vi "FRIC_navX_Get_RawValues_GyroAccelMag.vi"(5 "Device Number":T1, 7 "Update":bool) -> (2 "Raw Values (out)":T2)   [LabVIEW 2016, in "navX Library.lvlib"]
doc: "This navX VI returns the raw values from the Gyro, Accel, and Mag sensors."
uses:
  navX Library.lvlib
  _TypeDefs/FRIC_navX_DeviceNumbersTypeDef.ctl
  _TypeDefs/Z900_navX_DeviceRegisters.ctl
  _Util/Z900_navX_Util_LittleEndian_to_BigEndian.vi
  _Internal/FRIC_navX_Get_Registry.vi
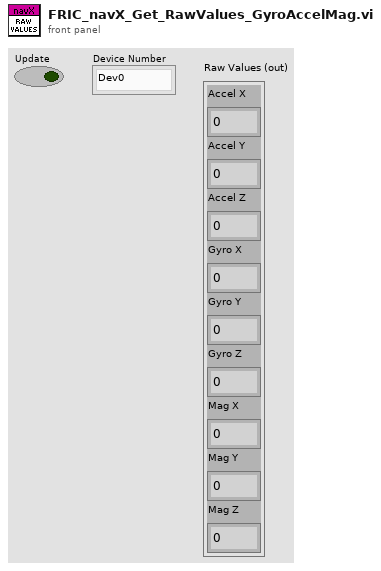
[diagram p1: front panel]
types:
  T1 = typedef "navX Library.lvlib/FRIC_navX_DeviceNumbersTypeDef.ctl" = enum16{"Dev0", "Dev1", "Dev2", "Dev3"}
  T2 = cluster{"Accel X":dbl, "Accel Y":dbl, "Accel Z":dbl, "Gyro X":dbl, "Gyro Y":dbl, "Gyro Z":dbl, "Mag X":dbl, "Mag Y":dbl, "Mag Z":dbl}
  T3 = typedef "navX Library.lvlib/Z900_navX_DeviceRegisters.ctl" = u8
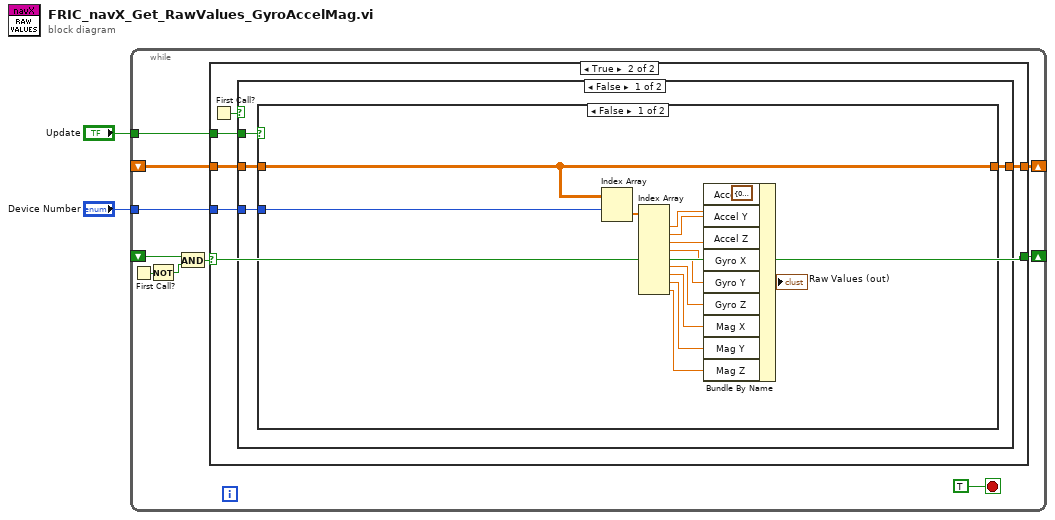
[diagram p0: block diagram]
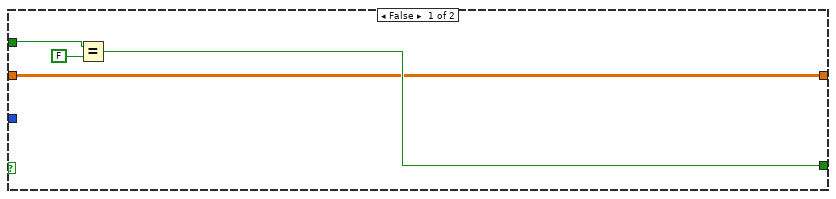
[diagram p2: hidden frame]
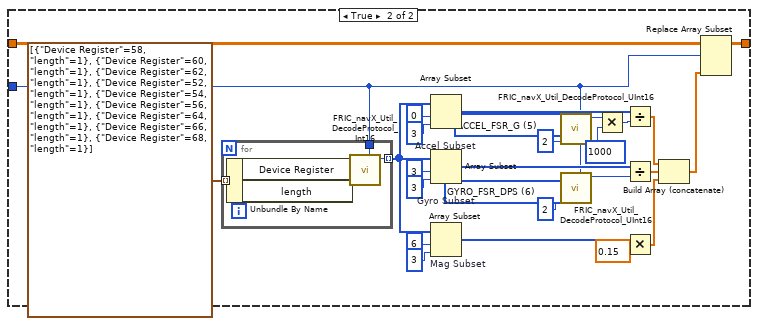
[diagram p3: hidden frame]
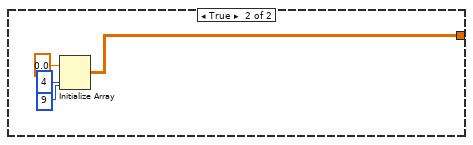
[diagram p4: hidden frame]
diagram:
  n1 = while {
    shift-right: [w12] -> _
    shift-left: _ -> [w9]
    tunnel: "Update" -> [w10]
    tunnel: "Device Number" -> [w8]
    shift-right: [w3] -> _
    shift-left: _ -> [w4]
    stop <- TRUE stop-if-true
    n2 = First Call?() -> (First Call?: T/F=w6:bool)
    n3 = Not(x=w6) -> (.not. x?=w7:bool)
    n4 = And(x=w4, y=w7) -> (x .and. y?=w5:bool)
    n5 = case shown="True" w5 {
      selector: w5 -> [_ w17]
      tunnel: [w13 w22] -> w12
      tunnel: w10 -> [w15 w21]
      tunnel: w9 -> [w13 w20]
      tunnel: w8 -> [_ w19]
      tunnel: [w14 w17] -> w3
      frame False {
        n6 = Equal?(x=w15, y=FALSE) -> (x = y?=w14:bool)
      }
      frame True {
        n7 = First Call?() -> (First Call?: T/F=w18:bool)
        n8 = case shown="False" w18 {
          tunnel: [w26 w75] -> w22
          tunnel: w21 -> [w25 _]
          tunnel: w20 -> [w24 _]
          tunnel: w19 -> [w23 _]
          frame False {
            n9 = case shown="False" w25 {
              tunnel: [w28 w43] -> w26
              tunnel: w24 -> [w28 w44]
              tunnel: w23 -> [w27 w42]
              frame False {
                n10 = Index Array(array=w28, index (row)=w27) -> (element=w29:dbl[])  [unwired: 1 in]
                n11 = Index Array(array=w29) -> (element #1=w31:dbl, element #2=w32:dbl, element #3=w33:dbl, element #4=w34:dbl, element #5=w35:dbl, element #6=w36:dbl, element #7=w37:dbl, element #8=w38:dbl, element #9=w39:dbl)  [unwired: 9 in]
                n12 = Bundle By Name(cluster=T2 {"Accel X"=0.0, "Accel Y"=0.0, "Accel Z"=0.0, "Gyro X"=0.0, "Gyro Y"=0.0, "Gyro Z"=0.0, "Mag X"=0.0, "Mag Y"=0.0, "Mag Z"=0.0}, "Accel X"=w31, "Accel Y"=w32, "Accel Z"=w33, "Gyro X"=w34, "Gyro Y"=w35, "Gyro Z"=w36, "Mag X"=w37, "Mag Y"=w38, "Mag Z"=w39) -> (→"Raw Values (out)":T2)
              }
              frame True {
                w48 = T3 5 items=["WHOAMI"=0, "HW_REV"=1, "FW_VER_MAJOR"=2, "FW_VER_MINOR"=3, "UPDATE_RATE_HZ"=4, "ACCEL_FSR_G"=5, "GYRO_FSR_DPS"=6, "OP_STATUS"=8, "CAL_STATUS"=9, "SELFTEST_STATUS"=10, "CAPABILITY_FLAGS_L"=11, "CAPABILITY_FLAGS_H"=12, "SENSOR_STATUS"=16, "TIMESTAMP"=18, "YAW"=22, "ROLL"=24, "PITCH"=26, "HEADING"=28, "FUSED_HEADING"=30, "ALTITUDE_I"=32, "ALTITUDE_D"=34, "LINERA_ACC_X"=36, "LINERA_ACC_Y"=38, "LINERA_ACC_Z"=40, "QUAT_W"=42, "QUAT_X"=44, "QUAT_Y"=46, "QUAT_Z"=48, "MPU_TEMP_C"=50, "GYRO_X"=52, "GYRO_Y"=54, "GYRO_Z"=56, "ACC_X"=58, "ACC_Y"=60, "ACC_Z"=62, "MAG_X"=64, "MAG_Y"=66, "MAG_Z"=68, "PRESSURE_I"=70, "PRESSURE_D"=72, "PRESSURE_TEMP"=74, "YAW_OFFSET"=76, "QUAT_OFFSET_W"=78, "QUAT_OFFSET_X"=80, "QUAT_OFFSET_Y"=82, "QUAT_OFFSET_Z"=84, "INTEGRATION_CONTROL"=86, "VELOCITY_X"=88, "VELOCITY_Y"=92, "VELOCITY_Z"=96, "DISPLACMENT_X"=100, "DISPLACMENT_Y"=104, "DISPLACEMENT_Z"=108] ("Device Register")
                w52 = T3 6 items=["WHOAMI"=0, "HW_REV"=1, "FW_VER_MAJOR"=2, "FW_VER_MINOR"=3, "UPDATE_RATE_HZ"=4, "ACCEL_FSR_G"=5, "GYRO_FSR_DPS"=6, "OP_STATUS"=8, "CAL_STATUS"=9, "SELFTEST_STATUS"=10, "CAPABILITY_FLAGS_L"=11, "CAPABILITY_FLAGS_H"=12, "SENSOR_STATUS"=16, "TIMESTAMP"=18, "YAW"=22, "ROLL"=24, "PITCH"=26, "HEADING"=28, "FUSED_HEADING"=30, "ALTITUDE_I"=32, "ALTITUDE_D"=34, "LINERA_ACC_X"=36, "LINERA_ACC_Y"=38, "LINERA_ACC_Z"=40, "QUAT_W"=42, "QUAT_X"=44, "QUAT_Y"=46, "QUAT_Z"=48, "MPU_TEMP_C"=50, "GYRO_X"=52, "GYRO_Y"=54, "GYRO_Z"=56, "ACC_X"=58, "ACC_Y"=60, "ACC_Z"=62, "MAG_X"=64, "MAG_Y"=66, "MAG_Z"=68, "PRESSURE_I"=70, "PRESSURE_D"=72, "PRESSURE_TEMP"=74, "YAW_OFFSET"=76, "QUAT_OFFSET_W"=78, "QUAT_OFFSET_X"=80, "QUAT_OFFSET_Y"=82, "QUAT_OFFSET_Z"=84, "INTEGRATION_CONTROL"=86, "VELOCITY_X"=88, "VELOCITY_Y"=92, "VELOCITY_Z"=96, "DISPLACMENT_X"=100, "DISPLACMENT_Y"=104, "DISPLACEMENT_Z"=108] ("Device Register")
                n13 = for {
                  tunnel: cluster{"Device Register":T3, "length":i32}[] [{"Device Register"=58, "length"=1}, {"Device Register"=60, "length"=1}, {"Device Register"=62, "length"=1}, {"Device Register"=52, "length"=1}, {"Device Register"=54, "length"=1}, {"Device Register"=56, "length"=1}, {"Device Register"=64, "length"=1}, {"Device Register"=66, "length"=1}, {"Device Register"=68, "length"=1}] ("Array") -> [w70] mode=indexing
                  tunnel: [w69] -> w45 mode=indexing
                  tunnel: w42 -> [w68]
                  n14 = Unbundle By Name(w70) -> ("Device Register"=w72:T3, "length"=w71:i32)
                  n15 = call "FRIC_navX_Util_DecodeProtocol_Int16.vi"("Device Number"=w68, "length"=w71, "Device Register"=w72) -> ("Value"=w69:i16)  [unwired: 8 in]
                }
                n16 = Array Subset "Accel Subset"(array=w45, index=0, length=3) -> (w61:i16[])
                n17 = Array Subset "Gyro Subset"(array=w45, index=3, length=3) -> (w60:i16[])
                n18 = Array Subset "Mag Subset"(array=w45, index=6, length=3) -> (w58:i16[])
                n19 = call "FRIC_navX_Util_DecodeProtocol_UInt16.vi"("Device Number"=w42, "length"=2, "Device Register"=w48) -> ("Value"=w46:u16)  [unwired: 8 in]
                n20 = call "FRIC_navX_Util_DecodeProtocol_UInt16.vi"("Device Number"=w42, "length"=2, "Device Register"=w52) -> ("Value"=w50:u16)  [unwired: 8 in]
                n21 = Multiply(x=w46, y=u16 1000) -> (x*y=w53:u16)
                n22 = Divide(x=w61, y=w53) -> (x/y=w57:dbl[])
                n23 = Divide(x=w60, y=w50) -> (x/y=w56:dbl[])
                n24 = Multiply(x=w58, y=0.15) -> (x*y=w55:dbl[])
                n25 = Build Array (concatenate)(w57, w56, w55) -> (w41:dbl[])
                n26 = Replace Array Subset(array=w44, new element=w41, index (row)=w42) -> (w43:dbl[][])  [unwired: 1 in]
              }
            }
          }
          frame True {
            n27 = Initialize Array(0.0, 4 ("dimension size"), 9 ("dimension size")) -> (w75:dbl[][])
          }
        }
      }
    }
  }
